vi "Read.vi"(11 "ConfigInfoValue in":refnum<class "ConfigInfoValue.lvclass">) -> (2 "Config Info":T1)   [LabVIEW 2020, in "Volatus.lvlib" / "ConfigInfoValue.lvclass"]
uses:
  ConfigInfoValue.lvclass
  ConfigInfoValue.lvclass/ConfigInfoValue.ctl
  Config Info.ctl
  Volatus.lvlib
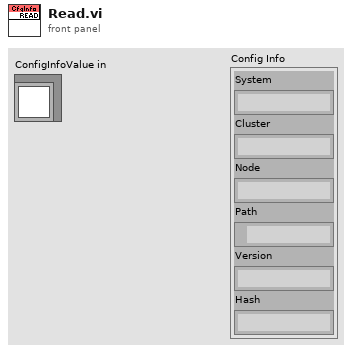
[diagram p1: front panel]
types:
  T1 = typedef "Volatus.lvlib/Config Info.ctl" = cluster{"System":string, "Cluster":string, "Node":string, "Path":path, "Version":string, "Hash":string}
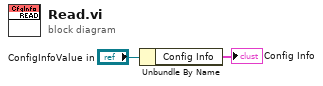
[diagram p0: block diagram]
diagram:
  n1 = Unbundle By Name("ConfigInfoValue in") -> ("Config Info"=→"Config Info":T1)
